vi "Append Data.vi"(8 "error in (no error)":errorcluster, 9 "Data":variant, 10 "ParamTags":T1, 11 "Rigol DG822 Sine in":refnum<class "Rigol DG822 Sine.lvclass">) -> (0 "error out":errorcluster, 3 "Rigol DG822 Sine out":refnum<class "Rigol DG822 Sine.lvclass">)   [LabVIEW 2021, in "Rigol DG822 UI.lvlib" / "Rigol DG822 Sine.lvlib" / "Rigol DG822 Sine.lvclass"]
uses:
  Rigol DG822 Sine.lvclass
  Rigol DG822 UI/lib/controls.llb/WaveformParamTags.ctl
  Rigol DG822 UI/lib/controls.llb/PeriodUnit.ctl
  Rigol DG822 Sine.lvclass/Rigol DG822 Sine.ctl
  Rigol DG822 UI/lib/controls.llb/FreqUnit.ctl
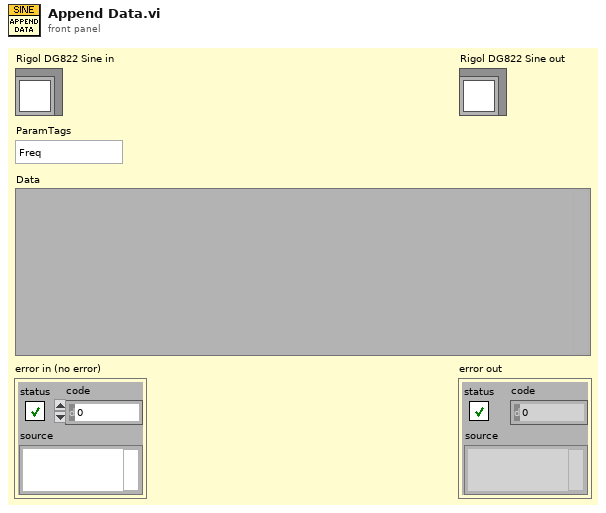
[diagram p1: front panel]
types:
  T1 = typedef "WaveformParamTags.ctl" = enum16{"Freq", "Period", "Ampl", "HighL", "Offset", "LowL", "Phase", "Duty", "Width", "RisEdge", "FallEdge"}
  T2 = cluster{"Freq":dbl, "FreqUnit":enum32{"No Selection", "MHz", "kHz", "Hz", "mHz", "uHz"}, "FreqUnitPrcs":dbl}
  T3 = typedef "PeriodUnit.ctl" = enum32{"No Selection", "s", "ms", "us", "ns"}
  T4 = cluster{"Period":dbl, "PeriodUnit":enum32{"No Selection", "s", "ms", "us", "ns"}, "PeriodUnitPrcs":dbl}
  T5 = typedef "FreqUnit.ctl" = enum32{"No Selection", "MHz", "kHz", "Hz", "mHz", "uHz"}
  T6 = cluster{"Offset":dbl, "OffsetUnit":enum32{"No Selection", "Vdc", "mVdc"}, "OffsetUnitPrecision":dbl}
  T7 = cluster{"Ampl":dbl, "AmplUnit":enum32{"No Selection", "Vpp", "mVpp"}, "AmplUnitPrecision":dbl}
  T8 = cluster{"HighL":dbl, "HighLUnit":enum32{"No Selection", "V", "mV"}, "HighLUnitPrcs":dbl}
  T9 = cluster{"Offset":dbl, "OffsetUnit":enum32{"No Selection", "Vdc", "mVdc"}, "OffsetUnitPrcs":dbl}
  T10 = cluster{"LowL":dbl, "LowLUnit":enum32{"No Selection", "V", "mV"}, "LowLUnitPrcs":dbl}
  T11 = cluster{"Phase":dbl, "PhaseUnit":enum32{"°"}, "PhaseUnitPrecision":dbl}
  T12 = enum32{"No Selection", "MHz", "kHz", "Hz", "mHz", "uHz"}
  T13 = cluster{dbl, "HighLUnit":enum32{"No Selection", "V", "mV"}, dbl}
  T14 = cluster{"Offset":dbl, "OffsetUnit":enum32{"No Selection", "Vdc", "mVdc"}, dbl}
  T15 = cluster{dbl, "AmplUnit":enum32{"No Selection", "Vpp", "mVpp"}, dbl}
  T16 = cluster{"LowL":dbl, "OffsetUnit":enum32{"No Selection", "Vdc", "mVdc"}, dbl}
  T17 = cluster{"LowL":dbl, "HighLUnit":enum32{"No Selection", "V", "mV"}, dbl}
  T18 = cluster{"Ampl":dbl, "AmplUnit":enum32{"No Selection", "Vpp", "mVpp"}, dbl}
  T19 = cluster{"HighL":dbl, "OffsetUnit":enum32{"No Selection", "Vdc", "mVdc"}, dbl}
  T20 = cluster{"HighL":dbl, "HighLUnit":enum32{"No Selection", "V", "mV"}, dbl}
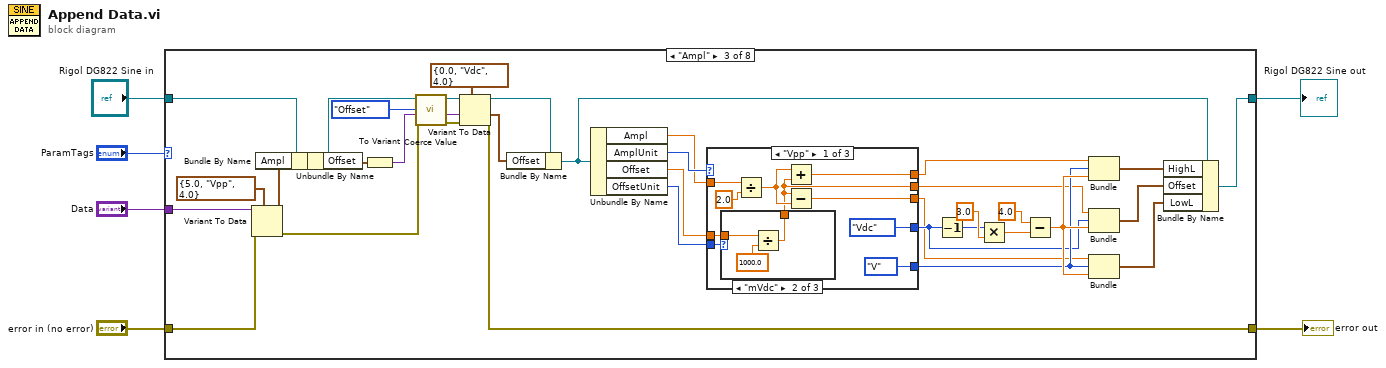
[diagram p0: block diagram]
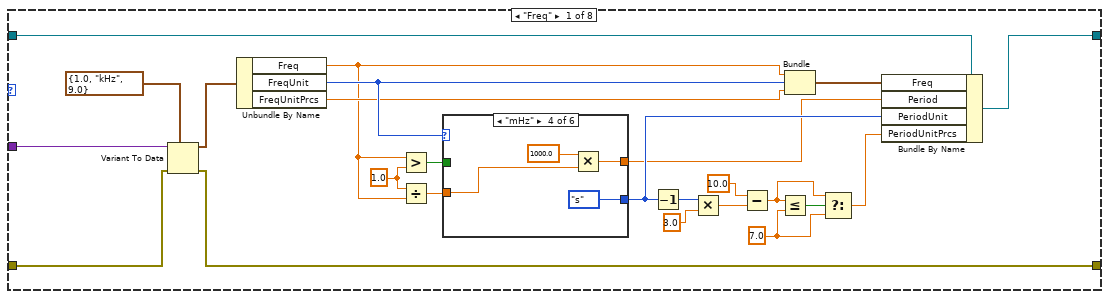
[diagram p2: hidden frame]
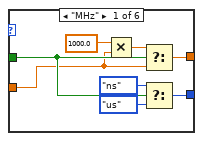
[diagram p3: hidden frame]
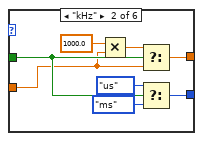
[diagram p4: hidden frame]
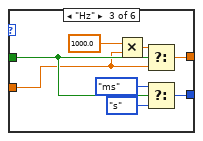
[diagram p5: hidden frame]
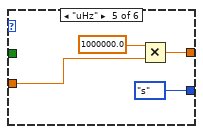
[diagram p6: hidden frame]
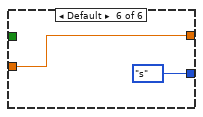
[diagram p7: hidden frame]
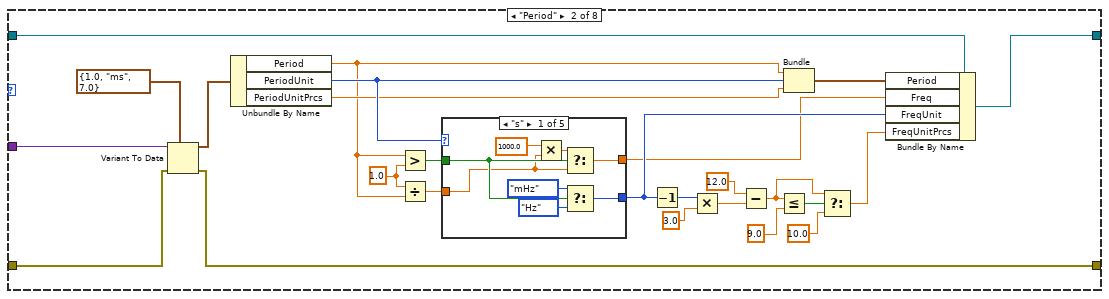
[diagram p8: hidden frame]
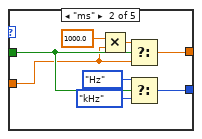
[diagram p9: hidden frame]
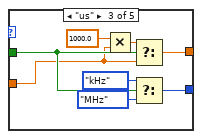
[diagram p10: hidden frame]
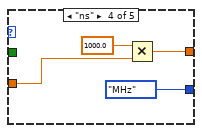
[diagram p11: hidden frame]
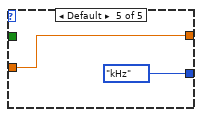
[diagram p12: hidden frame]
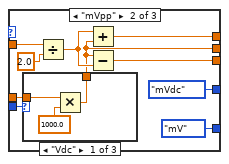
[diagram p15: hidden frame]
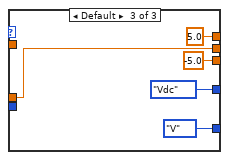
[diagram p18: hidden frame]
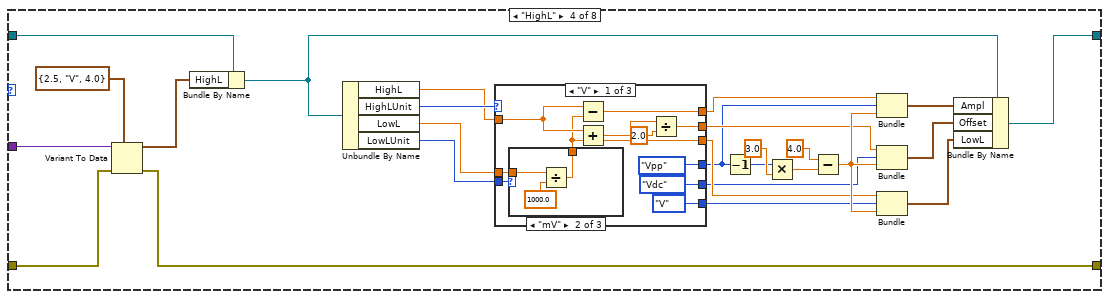
[diagram p19: hidden frame]
diagram:
  n1 = case shown="\"Ampl\"" "ParamTags" {
    tunnel: [w18 w69 w153 w214 w277 w338 w378 w386] -> w6
    tunnel: "error in (no error)" -> [w10 w67 w152 w213 w276 w337 w383 w385]
    tunnel: [w9 w66 w127 w212 w275 w336 w382 w385] -> w4
    tunnel: "Data" -> [w12 w71 w154 w215 w278 w339 w384 _]
    tunnel: "Rigol DG822 Sine in" -> [w8 w70 w129 w196 w258 w320 w379 w386]
    frame "Freq" {
      w22 = 7.0 ("y")
      w13 = 1.0 ("y")
      n2 = Variant To Data(error in=w10, type=T2 {"Freq"=1.0, "FreqUnit"=enum."kHz", "FreqUnitPrcs"=9.0} ("Freq"), Variant=w12) -> (data=w11:T2, error out=w9:errorcluster)
      n3 = Unbundle By Name(w11) -> ("Freq"=w14:dbl, "FreqUnit"=w17:T12, "FreqUnitPrcs"=w16:dbl)
      n4 = Greater?(x=w14, y=w13) -> (0:w27:bool)
      n5 = Divide(x=w13, y=w14) -> (x/y=w26:dbl)
      n6 = case shown="\"mHz\"" w17 {
        tunnel: [w38 w41 w51 PeriodUnit."s" ("f") PeriodUnit."s" ("f") PeriodUnit."s" ("f")] -> w29
        tunnel: w26 -> [w33 w43 w49 w55 w60 w63]
        tunnel: [w37 w42 w52 w58 w61 w63] -> w28
        tunnel: w27 -> [w36 w44 w50 _ _ _]
        frame "MHz" {
          n7 = Multiply(x=1000.0 ("y"), y=w33) -> (x*y=w35:dbl)
          n8 = Select(t=w35, s=w36, f=w33) -> (s? t:f=w37:dbl)
          n9 = Select(t=PeriodUnit."ns" ("PeriodUnit"), s=w36, f=PeriodUnit."us") -> (s? t:f=w38:T3)
        }
        frame "kHz" {
          n10 = Multiply(x=1000.0 ("y"), y=w43) -> (x*y=w46:dbl)
          n11 = Select(t=w46, s=w44, f=w43) -> (s? t:f=w42:dbl)
          n12 = Select(t=PeriodUnit."us" ("PeriodUnit"), s=w44, f=PeriodUnit."ms") -> (s? t:f=w41:T3)
        }
        frame "Hz" {
          n13 = Multiply(x=1000.0 ("y"), y=w49) -> (x*y=w54:dbl)
          n14 = Select(t=w54, s=w50, f=w49) -> (s? t:f=w52:dbl)
          n15 = Select(t=PeriodUnit."ms" ("f"), s=w50, f=PeriodUnit."s") -> (s? t:f=w51:T3)
        }
        frame "mHz" {
          n16 = Multiply(x=1000.0 ("y"), y=w55) -> (x*y=w58:dbl)
        }
        frame "uHz" {
          n17 = Multiply(x=1000000.0 ("y"), y=w60) -> (x*y=w61:dbl)
        }
        frame Default {
        }
      }
      n18 = Decrement(x=w29) -> (x-1=w30:T3)
      n19 = Multiply(x=w30, y=3.0) -> (x*y=w25:dbl)
      n20 = Subtract(x=10.0, y=w25) -> (x-y=w23:dbl)
      n21 = Less Or Equal?(x=w23, y=w22) -> (x <= y?=w24:bool)
      n22 = Bundle("Freq"=w14, "FreqUnit"=w17, "FreqUnitPrcs"=w16) -> (w19:T2)  [unwired: 1 in]
      n23 = Select(t=w23, s=w24, f=w22) -> (s? t:f=w15:dbl)
      n24 = Bundle By Name(cluster=w8, "Freq"=w19, "Period"=w28, "PeriodUnit"=w29, "PeriodUnitPrcs"=w15) -> (w18:refnum<class "Rigol DG822 Sine.lvclass">)
    }
    frame "Period" {
      w72 = 1.0 ("y")
      n25 = Variant To Data(error in=w67, type=T4 {"Period"=1.0, "PeriodUnit"=enum."ms", "PeriodUnitPrcs"=7.0} ("Period"), Variant=w71) -> (data=w68:T4, error out=w66:errorcluster)
      n26 = Unbundle By Name(w68) -> ("Period"=w73:dbl, "PeriodUnit"=w86:enum32{"No Selection", "s", "ms", "us", "ns"}, "PeriodUnitPrcs"=w75:dbl)
      n27 = Greater?(x=w73, y=w72) -> (0:w84:bool)
      n28 = Divide(x=w72, y=w73) -> (x/y=w85:dbl)
      n29 = case shown="\"s\"" w86 {
        tunnel: [w97 w102 w110 FreqUnit."MHz" ("FreqUnit") FreqUnit."kHz" ("FreqUnit")] -> w88
        tunnel: w85 -> [w92 w98 w106 w114 w118]
        tunnel: [w96 w103 w111 w117 w118] -> w87
        tunnel: w84 -> [w95 w99 w107 _ _]
        frame "s" {
          n30 = Multiply(x=1000.0 ("y"), y=w92) -> (x*y=w94:dbl)
          n31 = Select(t=w94, s=w95, f=w92) -> (s? t:f=w96:dbl)
          n32 = Select(t=FreqUnit."mHz" ("FreqUnit"), s=w95, f=FreqUnit."Hz") -> (s? t:f=w97:T5)
        }
        frame "ms" {
          n33 = Multiply(x=1000.0 ("y"), y=w98) -> (x*y=w105:dbl)
          n34 = Select(t=w105, s=w99, f=w98) -> (s? t:f=w103:dbl)
          n35 = Select(t=FreqUnit."Hz", s=w99, f=FreqUnit."kHz" ("FreqUnit")) -> (s? t:f=w102:T5)
        }
        frame "us" {
          n36 = Multiply(x=1000.0 ("y"), y=w106) -> (x*y=w113:dbl)
          n37 = Select(t=w113, s=w107, f=w106) -> (s? t:f=w111:dbl)
          n38 = Select(t=FreqUnit."kHz", s=w107, f=FreqUnit."MHz" ("FreqUnit")) -> (s? t:f=w110:T5)
        }
        frame "ns" {
          n39 = Multiply(x=1000.0 ("y"), y=w114) -> (x*y=w117:dbl)
        }
        frame Default {
        }
      }
      n40 = Decrement(x=w88) -> (x-1=w83:T5)
      n41 = Multiply(x=w83, y=3.0) -> (x*y=w82:dbl)
      n42 = Subtract(x=12.0, y=w82) -> (x-y=w80:dbl)
      n43 = Less Or Equal?(x=w80, y=9.0) -> (x <= y?=w81:bool)
      n44 = Bundle("Period"=w73, "PeriodUnit"=w86, "PeriodUnitPrcs"=w75) -> (w76:T4)  [unwired: 1 in]
      n45 = Select(t=w80, s=w81, f=10.0 ("y")) -> (s? t:f=w74:dbl)
      n46 = Bundle By Name(cluster=w70, "Period"=w76, "Freq"=w87, "FreqUnit"=w88, "FreqUnitPrcs"=w74) -> (w69:refnum<class "Rigol DG822 Sine.lvclass">)
    }
    frame "Ampl" {
      n47 = Variant To Data(error in=w152, type=T7 {"Ampl"=5.0, "AmplUnit"=enum."Vpp", "AmplUnitPrecision"=4.0} ("Ampl"), Variant=w154) -> (data=w130:T7, error out=w125:errorcluster)
      n48 = Bundle By Name(cluster=w129, "Ampl"=w130) -> (w128:refnum<class "Rigol DG822 Sine.lvclass">)
      n49 = Unbundle By Name(w128) -> ("Offset"=w150:T9)
      n50 = To Variant(anything=w150) -> (Variant=w124:variant)
      n51 = call-dynamic "Coerce Value.vi"("error in (no error)"=w125, "Value"=w124, "ParamTags"=WaveformParamTags."Offset", "Rigol DG822 Sine in"=w128) -> ("error out"=w126:errorcluster, "Coerced Value"=w146:variant, "Rigol DG822 Sine out"=w148:refnum<class "Rigol DG822 Sine.lvclass">)  [unwired: 5 in]
      n52 = Variant To Data(error in=w126, type=T6 {"Offset"=0.0, "OffsetUnit"=enum."Vdc", "OffsetUnitPrecision"=4.0} ("Offset"), Variant=w146) -> (data=w145:T6, error out=w127:errorcluster)
      n53 = Bundle By Name(cluster=w148, "Offset"=w145) -> (w131:refnum<class "Rigol DG822 Sine.lvclass">)
      n54 = Unbundle By Name(w131) -> ("Ampl"=w120:dbl, "AmplUnit"=w121:enum32{"No Selection", "Vpp", "mVpp"}, "Offset"=w122:dbl, "OffsetUnit"=w123:enum32{"No Selection", "Vdc", "mVdc"})
      n55 = case shown="\"Vpp\"" w121 {
        tunnel: [enum32{"No Selection", "Vdc", "mVdc"}."Vdc" ("OffsetUnit") enum32{"No Selection", "Vdc", "mVdc"}."mVdc" ("OffsetUnit") enum32{"No Selection", "Vdc", "mVdc"}."Vdc" ("OffsetUnit")] -> w135
        tunnel: w123 -> [w162 w177 _]
        tunnel: [enum32{"No Selection", "V", "mV"}."V" ("HighLUnit") enum32{"No Selection", "V", "mV"}."mV" ("HighLUnit") enum32{"No Selection", "V", "mV"}."V" ("HighLUnit")] -> w136
        tunnel: w120 -> [w160 w175 _]
        tunnel: w122 -> [w161 w176 w187]
        tunnel: [w157 w172 5.0] -> w134
        tunnel: [w156 w171 -5.0] -> w133
        tunnel: [w155 w170 w187] -> w132
        frame "Vpp" {
          n56 = case shown="\"mVdc\"" w162 {
            tunnel: w161 -> [w165 w168 w169]
            tunnel: [w165 w167 w169] -> w155
            frame "Vdc" {
            }
            frame "mVdc" {
              n57 = Divide(x=w168, y=1000.0) -> (x/y=w167:dbl)
            }
            frame Default {
            }
          }
          n58 = Divide(x=w160, y=2.0) -> (x/y=w158:dbl)
          n59 = Add(x=w158, y=w155) -> (x+y=w157:dbl)
          n60 = Subtract(x=w155, y=w158) -> (x-y=w156:dbl)
        }
        frame "mVpp" {
          n61 = case shown="\"Vdc\"" w177 {
            tunnel: w176 -> [w182 w183 w184]
            tunnel: [w181 w183 w184] -> w170
            frame "Vdc" {
              n62 = Multiply(x=w182, y=1000.0) -> (x*y=w181:dbl)
            }
            frame "mVdc" {
            }
            frame Default {
            }
          }
          n63 = Divide(x=w175, y=2.0) -> (x/y=w173:dbl)
          n64 = Add(x=w173, y=w170) -> (x+y=w172:dbl)
          n65 = Subtract(x=w170, y=w173) -> (x-y=w171:dbl)
        }
        frame Default {
        }
      }
      n66 = Decrement(x=w135) -> (x-1=w141:enum32{"No Selection", "Vdc", "mVdc"})
      n67 = Multiply(x=w141, y=3.0) -> (x*y=w142:dbl)
      n68 = Subtract(x=4.0, y=w142) -> (x-y=w137:dbl)
      n69 = Bundle(w134, "HighLUnit"=w136, w137) -> (w140:T13)  [unwired: 1 in]
      n70 = Bundle("Offset"=w132, "OffsetUnit"=w135, w137) -> (w139:T14)  [unwired: 1 in]
      n71 = Bundle(w133, "HighLUnit"=w136, w137) -> (w138:T13)  [unwired: 1 in]
      n72 = Bundle By Name(cluster=w131, "HighL"=w140, "Offset"=w139, "LowL"=w138) -> (w153:refnum<class "Rigol DG822 Sine.lvclass">)
    }
    frame "HighL" {
      n73 = Variant To Data(error in=w213, type=T8 {"HighL"=2.5, "HighLUnit"=enum."V", "HighLUnitPrcs"=4.0} ("HighL"), Variant=w215) -> (data=w197:T8, error out=w212:errorcluster)
      n74 = Bundle By Name(cluster=w196, "HighL"=w197) -> (w195:refnum<class "Rigol DG822 Sine.lvclass">)
      n75 = Unbundle By Name(w195) -> ("HighL"=w191:dbl, "HighLUnit"=w192:enum32{"No Selection", "V", "mV"}, "LowL"=w199:dbl, "LowLUnit"=w198:enum32{"No Selection", "V", "mV"})
      n76 = case shown="\"V\"" w192 {
        tunnel: [enum32{"No Selection", "Vpp", "mVpp"}."Vpp" ("AmplUnit") enum32{"No Selection", "Vpp", "mVpp"}."mVpp" ("AmplUnit") enum32{"No Selection", "Vpp", "mVpp"}."Vpp" ("AmplUnit")] -> w193
        tunnel: w198 -> [w225 w241 _]
        tunnel: [enum32{"No Selection", "V", "mV"}."V" ("HighLUnit") enum32{"No Selection", "V", "mV"}."mV" ("HighLUnit") enum32{"No Selection", "V", "mV"}."V" ("HighLUnit")] -> w203
        tunnel: w191 -> [w218 w233 _]
        tunnel: w199 -> [w224 w240 w252]
        tunnel: [w217 w232 5.0] -> w202
        tunnel: [w216 w234 -5.0] -> w201
        tunnel: [w220 w235 w252] -> w200
        tunnel: [enum32{"No Selection", "Vdc", "mVdc"}."Vdc" ("OffsetUnit") enum32{"No Selection", "Vdc", "mVdc"}."mVdc" ("OffsetUnit") enum32{"No Selection", "Vdc", "mVdc"}."Vdc" ("OffsetUnit")] -> w194
        frame "V" {
          n77 = case shown="\"mV\"" w225 {
            tunnel: w224 -> [w227 w230 w231]
            tunnel: [w227 w229 w231] -> w216
            frame "V" {
            }
            frame "mV" {
              n78 = Divide(x=w230, y=1000.0) -> (x/y=w229:dbl)
            }
            frame Default {
            }
          }
          n79 = Subtract(x=w218, y=w216) -> (x-y=w217:dbl)
          n80 = Add(x=w218, y=w216) -> (x+y=w219:dbl)
          n81 = Divide(x=w219, y=2.0) -> (x/y=w220:dbl)
        }
        frame "mV" {
          n82 = case shown="\"V\"" w241 {
            tunnel: w240 -> [w245 w246 w247]
            tunnel: [w244 w246 w247] -> w234
            frame "V" {
              n83 = Multiply(x=w245, y=1000.0) -> (x*y=w244:dbl)
            }
            frame "mV" {
            }
            frame Default {
            }
          }
          n84 = Subtract(x=w233, y=w234) -> (x-y=w232:dbl)
          n85 = Add(x=w233, y=w234) -> (x+y=w237:dbl)
          n86 = Divide(x=w237, y=2.0) -> (x/y=w235:dbl)
        }
        frame Default {
        }
      }
      n87 = Decrement(x=w193) -> (x-1=w208:enum32{"No Selection", "Vpp", "mVpp"})
      n88 = Multiply(x=w208, y=3.0) -> (x*y=w209:dbl)
      n89 = Subtract(x=4.0, y=w209) -> (x-y=w204:dbl)
      n90 = Bundle(w202, "AmplUnit"=w193, w204) -> (w207:T15)  [unwired: 1 in]
      n91 = Bundle("LowL"=w200, "OffsetUnit"=w194, w204) -> (w206:T16)  [unwired: 1 in]
      n92 = Bundle("LowL"=w201, "HighLUnit"=w203, w204) -> (w205:T17)  [unwired: 1 in]
      n93 = Bundle By Name(cluster=w195, "Ampl"=w207, "Offset"=w206, "LowL"=w205) -> (w214:refnum<class "Rigol DG822 Sine.lvclass">)
    }
    frame "Offset" {
      n94 = Variant To Data(error in=w276, type=T9 {"Offset"=0.0, "OffsetUnit"=enum."Vdc", "OffsetUnitPrcs"=4.0} ("Offset"), Variant=w278) -> (data=w259:T9, error out=w275:errorcluster)
      n95 = Bundle By Name(cluster=w258, "Offset"=w259) -> (w255:refnum<class "Rigol DG822 Sine.lvclass">)
      n96 = Unbundle By Name(w255) -> ("Offset"=w256:dbl, "OffsetUnit"=w257:enum32{"No Selection", "Vdc", "mVdc"}, "Ampl"=w261:dbl, "AmplUnit"=w260:enum32{"No Selection", "Vpp", "mVpp"})
      n97 = case shown="\"mVdc\"" w257 {
        tunnel: [enum32{"No Selection", "Vpp", "mVpp"}."Vpp" ("AmplUnit") enum32{"No Selection", "Vpp", "mVpp"}."mVpp" ("AmplUnit") enum32{"No Selection", "Vpp", "mVpp"}."Vpp" ("AmplUnit")] -> w265
        tunnel: w260 -> [w287 w302 _]
        tunnel: [enum32{"No Selection", "V", "mV"}."V" ("HighLUnit") enum32{"No Selection", "V", "mV"}."mV" ("HighLUnit") enum32{"No Selection", "V", "mV"}."V" ("HighLUnit")] -> w266
        tunnel: w256 -> [w282 w297 _]
        tunnel: w261 -> [w286 w301 w312]
        tunnel: [w285 w300 5.0] -> w264
        tunnel: [w284 w299 -5.0] -> w263
        tunnel: [w279 w294 w312] -> w262
        frame "Vdc" {
          n98 = case shown="\"Vpp\"" w287 {
            tunnel: w286 -> [w289 w292 w293]
            tunnel: [w289 w291 w293] -> w279
            frame "Vpp" {
            }
            frame "mVpp" {
              n99 = Divide(x=w292, y=1000.0) -> (x/y=w291:dbl)
            }
            frame Default {
            }
          }
          n100 = Divide(x=w279, y=2.0) -> (x/y=w281:dbl)
          n101 = Add(x=w282, y=w281) -> (x+y=w285:dbl)
          n102 = Subtract(x=w282, y=w281) -> (x-y=w284:dbl)
        }
        frame "mVdc" {
          n103 = case shown="\"Vpp\"" w302 {
            tunnel: w301 -> [w306 w307 w308]
            tunnel: [w305 w307 w308] -> w294
            frame "Vpp" {
              n104 = Multiply(x=w306, y=1000.0) -> (x*y=w305:dbl)
            }
            frame "mVpp" {
            }
            frame Default {
            }
          }
          n105 = Divide(x=w294, y=2.0) -> (x/y=w296:dbl)
          n106 = Add(x=w297, y=w296) -> (x+y=w300:dbl)
          n107 = Subtract(x=w297, y=w296) -> (x-y=w299:dbl)
        }
        frame Default {
        }
      }
      n108 = Decrement(x=w265) -> (x-1=w271:enum32{"No Selection", "Vpp", "mVpp"})
      n109 = Multiply(x=w271, y=3.0) -> (x*y=w272:dbl)
      n110 = Subtract(x=4.0, y=w272) -> (x-y=w267:dbl)
      n111 = Bundle(w264, "HighLUnit"=w266, w267) -> (w270:T13)  [unwired: 1 in]
      n112 = Bundle("Ampl"=w262, "AmplUnit"=w265, w267) -> (w269:T18)  [unwired: 1 in]
      n113 = Bundle(w263, "HighLUnit"=w266, w267) -> (w268:T13)  [unwired: 1 in]
      n114 = Bundle By Name(cluster=w255, "HighL"=w270, "Ampl"=w269, "LowL"=w268) -> (w277:refnum<class "Rigol DG822 Sine.lvclass">)
    }
    frame "LowL" {
      n115 = Variant To Data(error in=w337, type=T10 {"LowL"=-2.5, "LowLUnit"=enum."V", "LowLUnitPrcs"=4.0} ("LowL"), Variant=w339) -> (data=w321:T10, error out=w336:errorcluster)
      n116 = Bundle By Name(cluster=w320, "LowL"=w321) -> (w319:refnum<class "Rigol DG822 Sine.lvclass">)
      n117 = Unbundle By Name(w319) -> ("LowL"=w315:dbl, "LowLUnit"=w316:enum32{"No Selection", "V", "mV"}, "HighL"=w323:dbl, "HighLUnit"=w322:enum32{"No Selection", "V", "mV"})
      n118 = case shown="\"V\"" w316 {
        tunnel: [enum32{"No Selection", "Vpp", "mVpp"}."Vpp" ("AmplUnit") enum32{"No Selection", "Vpp", "mVpp"}."mVpp" ("AmplUnit") enum32{"No Selection", "Vpp", "mVpp"}."Vpp" ("AmplUnit")] -> w317
        tunnel: w322 -> [w349 w365 _]
        tunnel: [enum32{"No Selection", "V", "mV"}."V" ("HighLUnit") enum32{"No Selection", "V", "mV"}."mV" ("HighLUnit") enum32{"No Selection", "V", "mV"}."V" ("HighLUnit")] -> w327
        tunnel: w315 -> [w340 w356 _]
        tunnel: w323 -> [w348 w364 w376]
        tunnel: [w342 w358 5.0] -> w326
        tunnel: [w341 w357 -5.0] -> w325
        tunnel: [w344 w359 w376] -> w324
        tunnel: [enum32{"No Selection", "Vdc", "mVdc"}."Vdc" ("OffsetUnit") enum32{"No Selection", "Vdc", "mVdc"}."mVdc" ("OffsetUnit") enum32{"No Selection", "Vdc", "mVdc"}."Vdc" ("OffsetUnit")] -> w318
        frame "V" {
          n119 = case shown="\"V\"" w349 {
            tunnel: w348 -> [w351 w354 w355]
            tunnel: [w351 w353 w355] -> w341
            frame "V" {
            }
            frame "mV" {
              n120 = Divide(x=w354, y=1000.0) -> (x/y=w353:dbl)
            }
            frame Default {
            }
          }
          n121 = Subtract(x=w341, y=w340) -> (x-y=w342:dbl)
          n122 = Add(x=w340, y=w341) -> (x+y=w343:dbl)
          n123 = Divide(x=w343, y=2.0) -> (x/y=w344:dbl)
        }
        frame "mV" {
          n124 = case shown="\"V\"" w365 {
            tunnel: w364 -> [w369 w370 w371]
            tunnel: [w368 w370 w371] -> w357
            frame "V" {
              n125 = Multiply(x=w369, y=1000.0) -> (x*y=w368:dbl)
            }
            frame "mV" {
            }
            frame Default {
            }
          }
          n126 = Subtract(x=w357, y=w356) -> (x-y=w358:dbl)
          n127 = Add(x=w356, y=w357) -> (x+y=w361:dbl)
          n128 = Divide(x=w361, y=2.0) -> (x/y=w359:dbl)
        }
        frame Default {
        }
      }
      n129 = Decrement(x=w317) -> (x-1=w332:enum32{"No Selection", "Vpp", "mVpp"})
      n130 = Multiply(x=w332, y=3.0) -> (x*y=w333:dbl)
      n131 = Subtract(x=4.0, y=w333) -> (x-y=w328:dbl)
      n132 = Bundle(w326, "AmplUnit"=w317, w328) -> (w331:T15)  [unwired: 1 in]
      n133 = Bundle("HighL"=w324, "OffsetUnit"=w318, w328) -> (w330:T19)  [unwired: 1 in]
      n134 = Bundle("HighL"=w325, "HighLUnit"=w327, w328) -> (w329:T20)  [unwired: 1 in]
      n135 = Bundle By Name(cluster=w319, "Ampl"=w331, "Offset"=w330, "HighL"=w329) -> (w338:refnum<class "Rigol DG822 Sine.lvclass">)
    }
    frame "Phase" {
      n136 = Variant To Data(error in=w383, type=T11 {"Phase"=0.0, "PhaseUnit"=enum."°", "PhaseUnitPrecision"=3.0} ("Phase"), Variant=w384) -> (data=w380:T11, error out=w382:errorcluster)
      n137 = Bundle By Name(cluster=w379, "Phase"=w380) -> (w378:refnum<class "Rigol DG822 Sine.lvclass">)
    }
    frame Default {
    }
  }
  "error out" <- w4
  "Rigol DG822 Sine out" <- w6
